vi "LinearSmooth.vi"(1 "Smooth Length":i32=1, 2 "Array":dbl[](array[numeric])) -> (0 "Smoothed Array":dbl[](array[numeric]))   [LabVIEW 2010]
uses:
  <vilib>/Analysis/2dsp.llb/1D Convolution (DBL).vi
  <vilib>/Analysis/NI_AALPro.lvlib
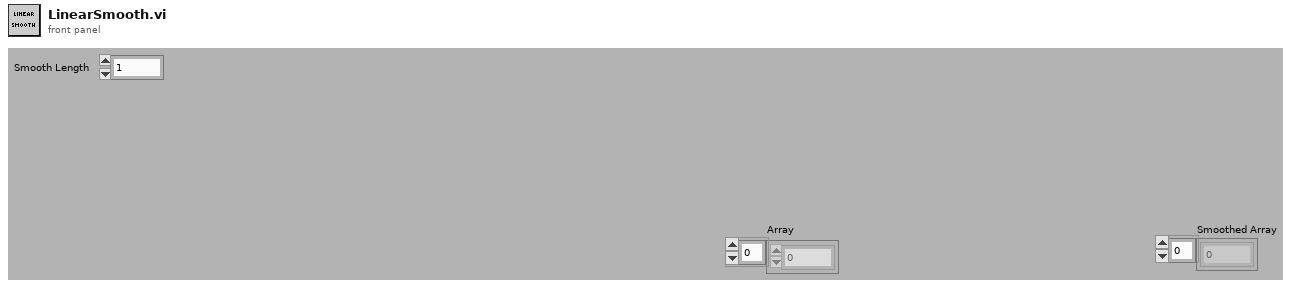
[diagram p1: front panel]
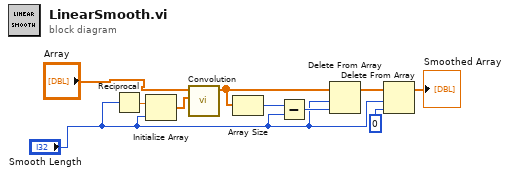
[diagram p0: block diagram]
diagram:
  n1 = Reciprocal(x="Smooth Length") -> (1/x=w4:dbl)
  n2 = Initialize Array(w4, "Smooth Length") -> (w5:dbl[])
  n3 = call-poly <vilib>:"Convolution.vi"("Y"=w5, "X"="Array") -> ("X * Y"=w7:dbl[])  [unwired: 8 in, 1 out]
  n4 = Array Size(array=w7) -> (size(s)=w8:i32)
  n5 = Subtract(x=w8, y="Smooth Length") -> (x-y=w9:i32)
  n6 = Delete From Array(array=w7, length="Smooth Length", index=w9) -> (array with subset deleted=w6:dbl[])  [unwired: 1 out]
  n7 = Delete From Array(array=w6, length="Smooth Length", index=0) -> (array with subset deleted=→"Smoothed Array":dbl[])  [unwired: 1 out]
